vi "crc.vi"(0 "Input string":string) -> (1 "Checksum (as hexadecimal)":string, 2 "Checksum (as string)":string)   [LabVIEW 2015]
doc: "moreChemistry's general purpose CRC vi\ncopyright 2004 moreChemistry BART BOSHUIZEN"
panel:
  in  "StartValue":i8
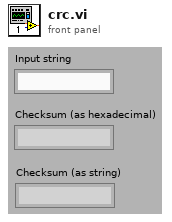
[diagram p1: front panel]
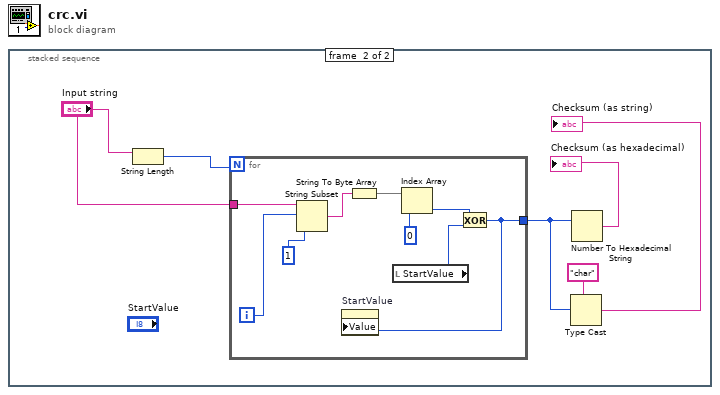
[diagram p0: block diagram]
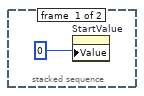
[diagram p2: hidden frame]
diagram:
  n1 = stacked-sequence {
    frame #0 {
      n2 = property on="StartValue" class="DigNum (strict)"("Value"=0) -> ()  [unwired: 2 in, 2 out]
    }
    frame #1 {
      n3 = String Length(string="Input string") -> (length=w7:i32)
      n4 = for {
        N: w7 -> [_]
        tunnel: "Input string" -> [w16]
        tunnel: [w9] -> w4
        i -> [w15]
        n5 = String Subset(string=w16, offset (0)=w15, length (rest)=1) -> (substring=w13:string)
        n6 = String To Byte Array(string=w13) -> (unsigned byte array=w8:u8[])
        n7 = local read "StartValue"() -> (w10:i8)
        n8 = Index Array(array=w8, index=0) -> (element=w12:u8)
        n9 = Exclusive Or(1:w10, 2:w12) -> (0:w9:u8)
        n10 = property on="StartValue" class="DigNum (strict)"("Value"=w9) -> ()  [unwired: 2 in, 2 out]
      }
      n11 = Type Cast(type="char", x=w4) -> (*(type *) &x=→"Checksum (as string)":string)
      n12 = Number To Hexadecimal String(2:w4) -> (0:→"Checksum (as hexadecimal)":string)  [unwired: 1 in]
    }
  }
